vi "Format_Extended_Write.vi"(0 "Source Address":u32=7, 2 "Address":u32=2, 5 "error in (no error)":errorcluster, 8 "BC":u32=1, 10 "Data_Blk_2":u32, 12 "Data_Blk_1":u32) -> (15 "RFFE Write Word":u32, 19 "error out":errorcluster)   [LabVIEW 2020, in "niDigital.lvclass"]
uses:
  niDigital.lvclass
panel:
  out "x << y 5":u32
  out "x << y 3":u32=15872
  out "x << y 2":u32=131072
  out "x << y":u32=491520
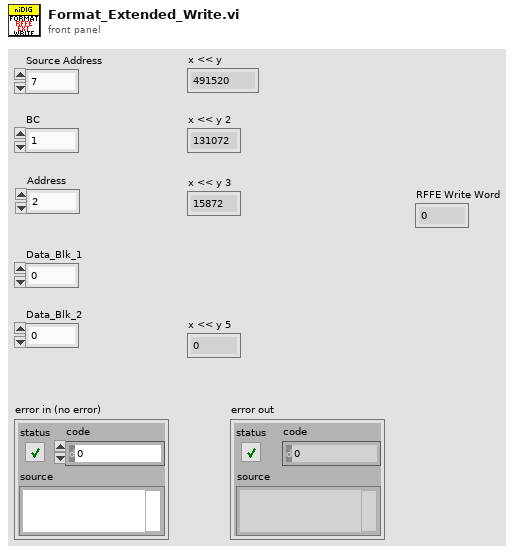
[diagram p1: front panel]
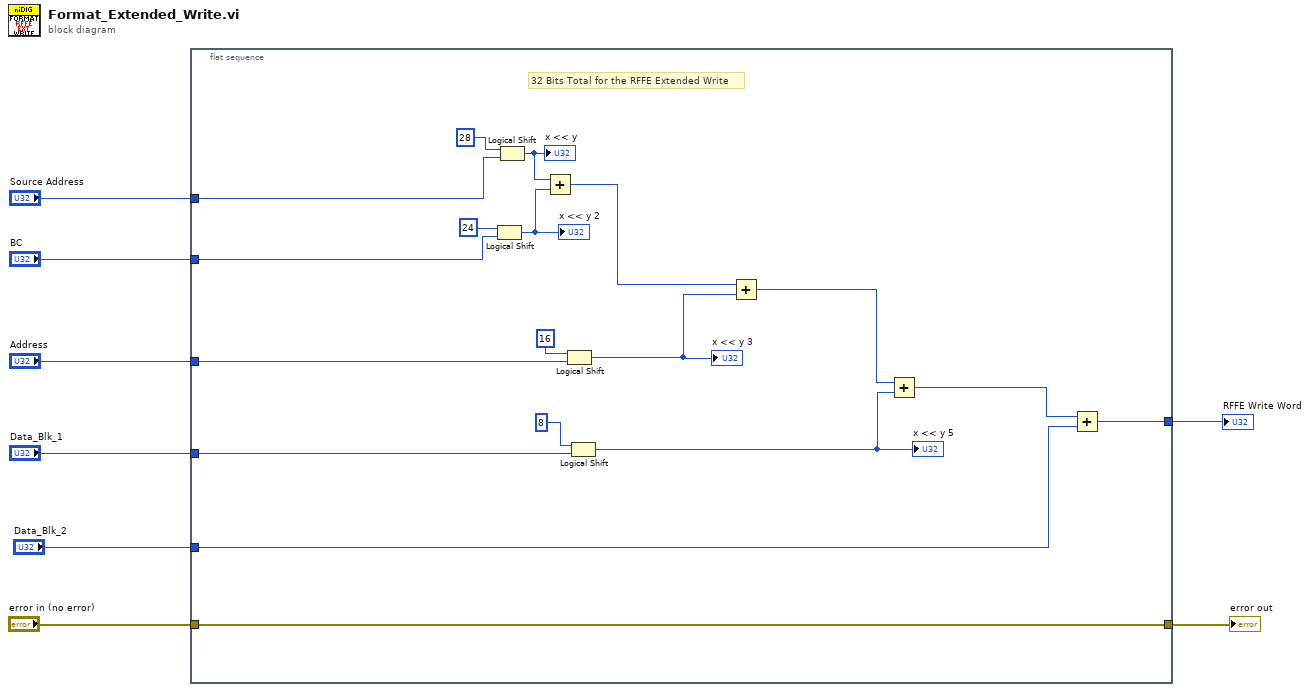
[diagram p0: block diagram]
diagram:
  n1 = flat-sequence {
    tunnel: "Source Address" -> [w26]
    tunnel: "BC" -> [w25]
    tunnel: "Address" -> [w24]
    tunnel: "Data_Blk_1" -> [w23]
    tunnel: "Data_Blk_2" -> [w9]
    tunnel: [w11] -> w3
    tunnel: [w10] -> w1
    tunnel: "error in (no error)" -> [w10]
    frame #0 {
      # "32 Bits Total for the RFFE Extended Write"
      n2 = Logical Shift(y=i16 24, x=w25) -> (x << y=w19:u32)
      "x << y 2" <- w19
      n3 = Logical Shift(y=i16 28, x=w26) -> (x << y=w21:u32)
      "x << y" <- w21
      n4 = Add(x=w21, y=w19) -> (x+y=w14:u32)
      n5 = Logical Shift(y=i16 16, x=w24) -> (x << y=w18:u32)
      "x << y 3" <- w18
      n6 = Logical Shift(y=i16 8, x=w23) -> (x << y=w15:u32)
      "x << y 5" <- w15
      n7 = Add(x=w14, y=w18) -> (x+y=w13:u32)
      n8 = Add(x=w13, y=w15) -> (x+y=w12:u32)
      n9 = Add(x=w12, y=w9) -> (x+y=w11:u32)
    }
  }
  "RFFE Write Word" <- w3
  "error out" <- w1
